vi "Helmholtz2D_FEM_Delaunay_Triangle.vi"(7 "init? (F)":bool, 8 "Triangles In":i32[][](array[numeric]), 9 "Index":i32[](array[numeric]), 10 "Y":dbl[](array[numeric]), 11 "X":dbl[](array[numeric])) -> (0 "Triangles Out":i32[][](array[numeric]), 1 "Edges":i32[][](array[numeric]), 2 "Y Out":dbl[](array[numeric]), 3 "X Out":dbl[](array[numeric]))   [LabVIEW 2017, in "NI_PDE.lvlib"]
uses:
  <vilib>/gmath/NI_PDE.lvlib
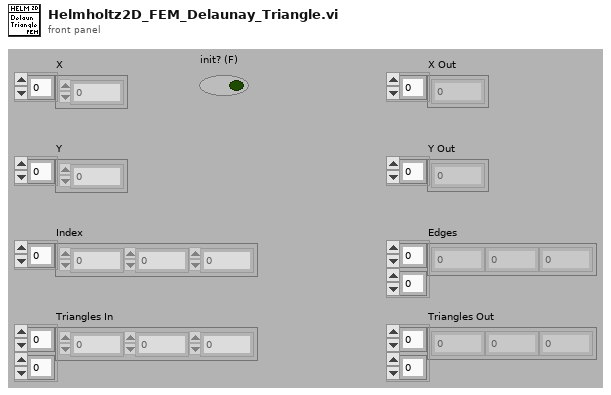
[diagram p1: front panel]
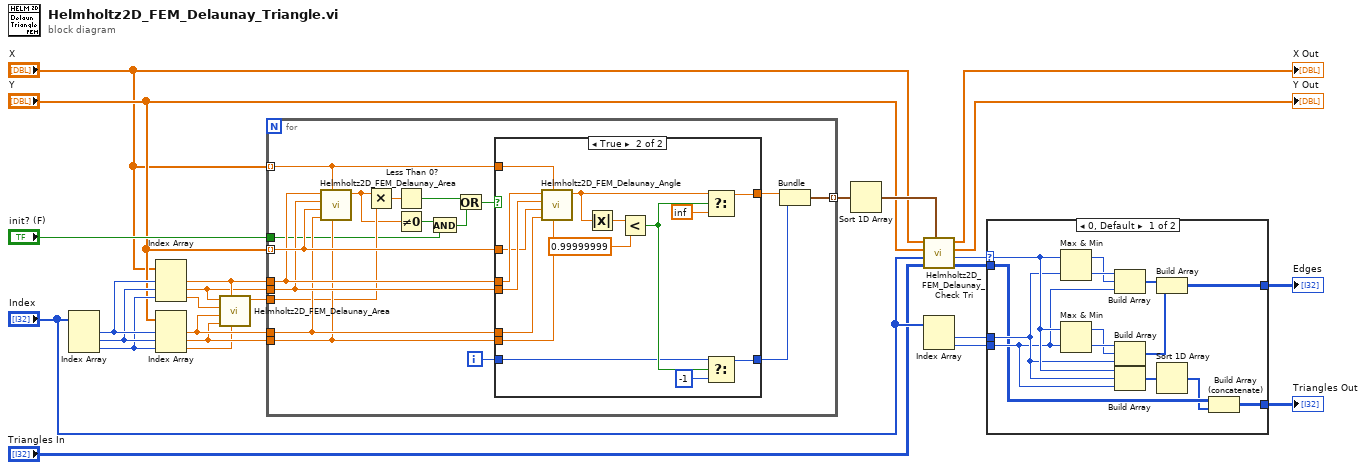
[diagram p0: block diagram]
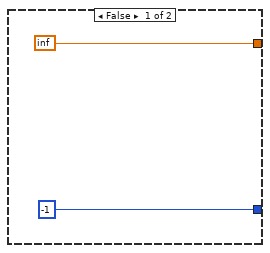
[diagram p3: hidden frame]
diagram:
  n1 = Index Array(array="Index") -> (element #1=w25:i32, element #2=w24:i32, element #3=w23:i32)  [unwired: 3 in]
  n2 = Index Array(array="X", index #1=w25, index #2=w24, index #3=w23) -> (element #1=w22:dbl, element #2=w21:dbl, element #3=w20:dbl)
  n3 = Index Array(array="Y", index #1=w25, index #2=w24, index #3=w23) -> (element #1=w19:dbl, element #2=w18:dbl, element #3=w17:dbl)
  n4 = call <vilib>:"Helmholtz2D_FEM_Delaunay_Area.vi"("y3"=w17, "x1"=w22, "y2"=w18, "y1"=w19, "x3"=w20, "x2"=w21) -> ("area"=w16:dbl)  [unwired: 5 out]
  n5 = for {
    tunnel: "X" -> [w42] mode=indexing
    tunnel: "Y" -> [w41] mode=indexing
    tunnel: w22 -> [w40]
    tunnel: w21 -> [w39]
    tunnel: w19 -> [w38]
    tunnel: w18 -> [w37]
    tunnel: w16 -> [w36]
    tunnel: "init? (F)" -> [w32]
    tunnel: [w26] -> w15 mode=indexing
    i -> [w43]
    n6 = call <vilib>:"Helmholtz2D_FEM_Delaunay_Area.vi"("y3"=w37, "x1"=w42, "y2"=w38, "y1"=w41, "x3"=w39, "x2"=w40) -> ("area"=w34:dbl)  [unwired: 5 out]
    n7 = Multiply(x=w34, y=w36) -> (x*y=w35:dbl)
    n8 = Less Than 0?(x=w35) -> (x < 0?=w31:bool)
    n9 = Not Equal To 0?(x=w34) -> (x != 0?=w33:bool)
    n10 = And(x=w33, y=w32) -> (x .and. y?=w30:bool)
    n11 = Or(x=w31, y=w30) -> (x .or. y?=w29:bool)
    n12 = case shown="True" w29 {
      tunnel: w43 -> [_ w48]
      tunnel: w42 -> [_ w60]
      tunnel: w41 -> [_ w57]
      tunnel: w40 -> [_ w59]
      tunnel: w39 -> [_ w58]
      tunnel: w38 -> [_ w56]
      tunnel: w37 -> [_ w55]
      tunnel: [inf w50] -> w28
      tunnel: [-1 ("y") w47] -> w27
      frame False {
      }
      frame True {
        n13 = call <vilib>:"Helmholtz2D_FEM_Delaunay_Angle.vi"("y3"=w55, "x1"=w60, "y2"=w56, "y1"=w57, "x3"=w58, "x2"=w59) -> ("angle"=w51:dbl)  [unwired: 5 out]
        n14 = Absolute Value(x=w51) -> (abs(x)=w54:dbl)
        n15 = Less?(x=w54, y=0.99999999) -> (x < y?=w49:bool)
        n16 = Select(t=w51, s=w49, f=inf) -> (s? t:f=w50:dbl)
        n17 = Select(t=w48, s=w49, f=-1) -> (s? t:f=w47:i32)
      }
    }
    n18 = Bundle("angle"=w28, "f"=w27) -> (w26:cluster{"angle":dbl, "f":i32})  [unwired: 1 out]
  }
  n19 = Sort 1D Array(array=w15) -> (sorted array=w14:cluster{"angle":dbl, "f":i32}[])
  n20 = call <vilib>:"Helmholtz2D_FEM_Delaunay_Check Tri.vi"("Angle"=w14, "Triangles In"="Triangles In", "Index"="Index", "Y"="Y", "X"="X") -> ("Triangles Out"=w10:i32[][], "new index"=w13:i32, "Y Out"=→"Y Out":dbl[], "X Out"=→"X Out":dbl[])  [unwired: 3 out]
  n21 = Index Array(array="Index") -> (element #1=w12:i32, element #2=w11:i32)  [unwired: 2 in]
  n22 = case shown="0, Default" w13 {
    selector: w13 -> [w67 _]
    tunnel: w11 -> [w65 _]
    tunnel: w12 -> [w66 _]
    tunnel: [w68 _] -> w7
    tunnel: w10 -> [w63 w75]
    tunnel: [w61 w75] -> w6
    frame 0, Default {
      n23 = Max & Min(x=w67, y=w66) -> (max(x,y)=w73:i32, min(x,y)=w74:i32)
      n24 = Max & Min(x=w67, y=w65) -> (max(x,y)=w71:i32, min(x,y)=w72:i32)
      n25 = Build Array(w74, w73, w65) -> (w70:i32[])
      n26 = Build Array(w72, w71, w66) -> (w69:i32[])
      n27 = Build Array(w67, w66, w65) -> (w64:i32[])
      n28 = Build Array(w70, w69) -> (w68:i32[][])
      n29 = Sort 1D Array(array=w64) -> (sorted array=w62:i32[])
      n30 = Build Array (concatenate)(w63, w62) -> (w61:i32[][])
    }
    frame ..-1 {
    }
  }
  "Edges" <- w7
  "Triangles Out" <- w6
